vi "Odometry2ROS.vi"(2 "OmniDynamics out":T1={"frame_id"="", "child_frame_id"="", "PoseCovariance"={"Pose"={"Point"={"x"=0.0, "y"=0.0, "z"=0.0}, "Quaternion"={"x"=0.0, "y"=0.0, "z"=0.0, "w"=0.0}}, "Covariance"=[0.0, 0.0, 0.0, 0.0, 0.0]}, "TwistCovariance"={"Twist"={"Linear"={"x"=0.0, "y"=0.0, "z"=0.0}, "Angular"={"x"=0.0, "y"=0.0, "z"=0.0}}, "Covariance"=[0.0, 0.0, 0.0, 0.0, 0.0]}}, 3 "msg in":string) -> (1 "msg out":string)   [LabVIEW 2014]
uses:
  Odometry.ctl
  TwistCovariance.ctl
  <userlib>/ROS for LabVIEW Software/ROS/MessageBuilding/std_msgs/subs/stringScalar.vi
  <userlib>/ROS for LabVIEW Software/ROS/MessageBuilding/std_msgs/subs/float64Array.vi
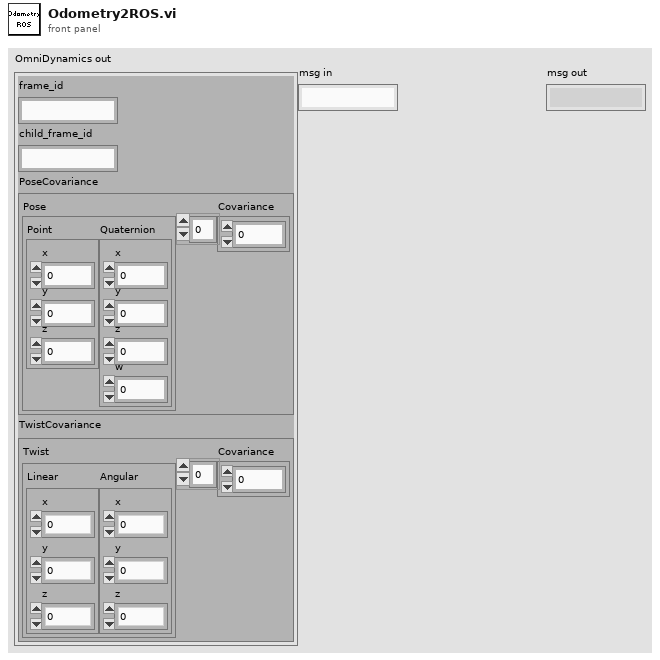
[diagram p1: front panel]
types:
  T1 = typedef "Odometry.ctl" = cluster{"frame_id":string, "child_frame_id":string, "PoseCovariance":cluster{"Pose":cluster{"Point":cluster{"x":dbl, "y":dbl, "z":dbl}, "Quaternion":cluster{"x":dbl, "y":dbl, "z":dbl, "w":dbl}}, "Covariance":dbl[]}, "TwistCovariance":T2}
  T2 = typedef "TwistCovariance.ctl" = cluster{"Twist":cluster{"Linear":cluster{"x":dbl, "y":dbl, "z":dbl}, "Angular":cluster{"x":dbl, "y":dbl, "z":dbl}}, "Covariance":dbl[]}
  T3 = cluster{"Pose":cluster{"Point":cluster{"x":dbl, "y":dbl, "z":dbl}, "Quaternion":cluster{"x":dbl, "y":dbl, "z":dbl, "w":dbl}}, "Covariance":dbl[]}
  T4 = cluster{"Linear":cluster{"x":dbl, "y":dbl, "z":dbl}, "Angular":cluster{"x":dbl, "y":dbl, "z":dbl}}
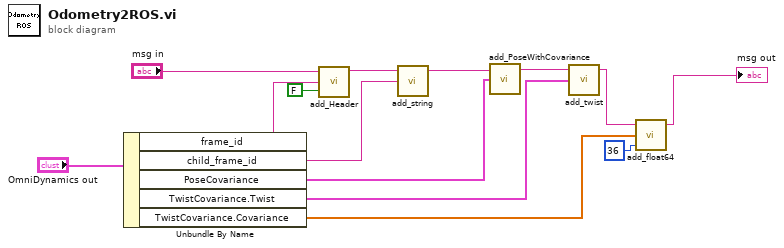
[diagram p0: block diagram]
diagram:
  n1 = Unbundle By Name("OmniDynamics out") -> ("frame_id"=w11:string, "child_frame_id"=w9:string, "PoseCovariance"=w7:T3, "TwistCovariance.Twist"=w4:T4, "TwistCovariance.Covariance"=w2:dbl[])
  n2 = call <userlib>:"add_Header.vi"("reset seq?"=FALSE, "frame_id"=w11, "msg in"="msg in") -> ("msg out"=w10:string)  [unwired: 2 in]
  n3 = call-poly <userlib>:"add_string.vi"("String"=w9, "msg in"=w10) -> ("msg out"=w8:string)  [unwired: 3 in]
  n4 = call <userlib>:"add_PoseWithCovariance.vi"("PoseCovariance"=w7, "msg in"=w8) -> ("msg out"=w5:string)  [unwired: 3 in]
  n5 = call <userlib>:"add_twist.vi"("Twist"=w4, "msg in"=w5) -> ("msg out"=w3:string)  [unwired: 3 in]
  n6 = call-poly <userlib>:"add_float64.vi"("Array Length"=36, "Array"=w2, "msg in"=w3) -> ("msg out"=→"msg out":string)  [unwired: 2 in]
